vi "SaveCSVImage.vi"(9 "Image":u16[][](array[numeric]), 10 "FileName":string, 11 "Path":path) -> ()   [LabVIEW 2023, in "InterferometryUI.lvlib" / "InterferometryUI.lvclass"]
uses:
  InterferometryUI.lvclass
  <vilib>/Utility/file.llb/Write Delimited Spreadsheet (I64).vi
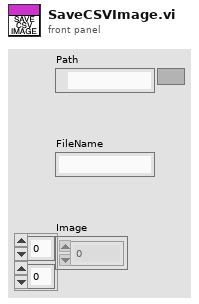
[diagram p1: front panel]
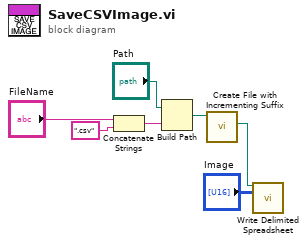
[diagram p0: block diagram]
diagram:
  n1 = Concatenate Strings("FileName", ".csv" ("string")) -> (w6:string)
  n2 = Build Path(base path="Path", name or relative path=w6) -> (appended path=w2:path)
  n3 = call <vilib>:"Create File with Incrementing Suffix.vi"("file path"=w2) -> ("actual path"=w3:path)  [unwired: 8 in, 2 out]
  n4 = call-poly <vilib>:"Write Delimited Spreadsheet.vi"("file path (dialog if empty)"=w3, "2D data"="Image") -> ()  [unwired: 12 in, 2 out]
